vi "dfd_FXP Direct IIR II with IS.vi"(6 "state in":i64[](array[numeric]), 7 "quantizers":T5[](array[typedef]) {"source" items=["Coef a/k"=0, "Coef b/v"=7, "Input"=1, "Output"=2, "Multiplicand"=3, "Product"=4, "Sum"=5, "Delay"=6, "Gain"=8]}, 8 "filtering statistics in":T4(array[cluster]) {"statistics information"."min value" format="%.2f"; "statistics information"."max value" format="%.2f"; "Quantizer Source" items=["Coefficients a/k"=0, "Coefficients b/v"=7, "Input"=1, "Output"=2, "Multiplicand"=3, "Product"=4, "Sum"=5, "Delay"=6]}, 9 "coef a":T7, 10 "coef b":T7, 11 "X":T7) -> (0 "filtering statistics out":T4(array[cluster]) {"statistics information"."min value" format="%.2f"; "statistics information"."max value" format="%.2f"; "Quantizer Source" items=["Coefficients a/k"=0, "Coefficients b/v"=7, "Input"=1, "Output"=2, "Multiplicand"=3, "Product"=4, "Sum"=5, "Delay"=6]}, 3 "filtered X":T7, 4 "state out":i64[](array[numeric]))   [LabVIEW 2017, in "NI_DigFilter_FXP.lvlib"]
uses:
  <vilib>/addons/Digital Filter Design/NI_DigFilter_FXP.lvlib
  <vilib>/addons/Digital Filter Design/_Objects.llb/dfd_DFXP Data Type (vector).ctl
  <vilib>/addons/Digital Filter Design/_Objects.llb/dfd_DFXP Operation Parameter.ctl
  <vilib>/addons/Digital Filter Design/_Objects.llb/dfd_Internal Quantization Srcs.ctl
  <vilib>/addons/Digital Filter Design/_Objects.llb/DFD Quantization Sources.ctl
  <vilib>/addons/Digital Filter Design/_Objects.llb/DFD FXP Statistics Data.ctl
  <vilib>/addons/Digital Filter Design/_Objects.llb/dfd_DFXP Data Type (scaler).ctl
  <vilib>/addons/Digital Filter Design/NI_DigFilterLicensed.lvlib
panel:
  in  "DFXP Value":T1={"value"=0, "wl"=0, "iwl"=0, "Signed"=TRUE} {"value" format="%.0x"}
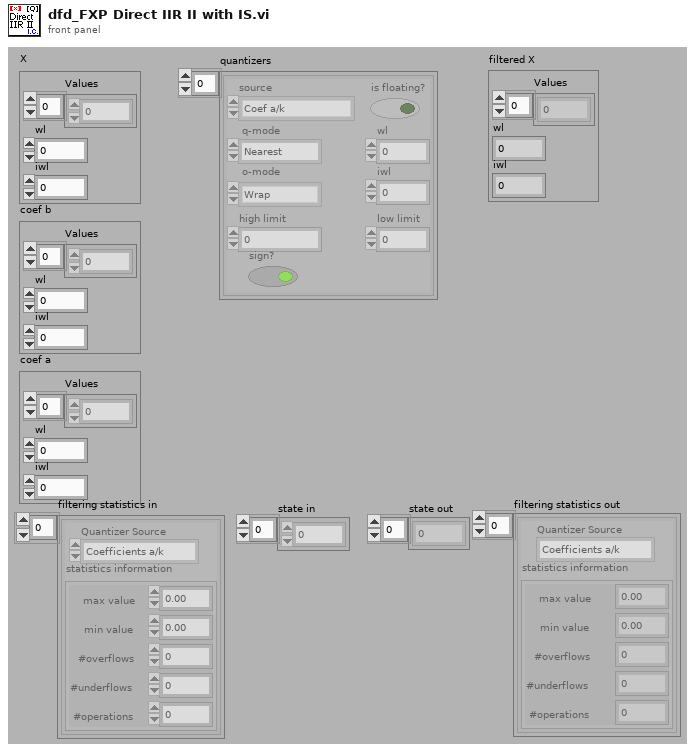
[diagram p1: front panel]
types:
  T1 = typedef "dfd_DFXP Data Type (scaler).ctl" = cluster{"value":i64, "wl":i16, "iwl":i16, "Signed":bool}
  T2 = typedef "NI_DigFilterLicensed.lvlib/DFD Quantization Sources.ctl" = u16
  T3 = typedef "NI_DigFilterLicensed.lvlib/DFD FXP Statistics Data.ctl" = cluster{"max value":ext, "min value":ext, "#overflows":i32, "#underflows":i32, "#operations":i32}
  T4 = cluster{"Quantizer Source":T2, "statistics information":T3}[]
  T5 = typedef "dfd_DFXP Operation Parameter.ctl" = cluster{"source":T6, "is floating?":bool, "o-mode":enum16{"Saturation", "Wrap"}, "q-mode":enum16{"Nearest", "Truncation"}, "wl":i16, "high limit":i64, "low limit":i64, "iwl":i16, "sign?":bool}
  T6 = typedef "NI_DigFilterLicensed.lvlib/dfd_Internal Quantization Srcs.ctl" = u16
  T7 = typedef "dfd_DFXP Data Type (vector).ctl" = cluster{"Values":i64[], "wl":i16, "iwl":i16}
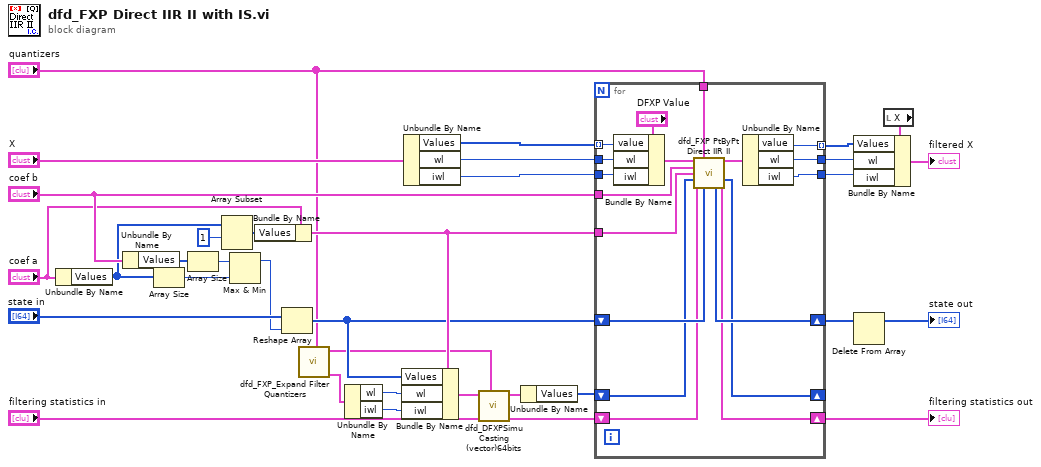
[diagram p0: block diagram]
diagram:
  n1 = Unbundle By Name("coef a") -> ("Values"=w21:i64[])
  n2 = Unbundle By Name("coef b") -> ("Values"=w22:i64[])
  n3 = Array Size(array=w21) -> (size(s)=w32:i32)
  n4 = Array Size(array=w22) -> (size(s)=w31:i32)
  n5 = Array Subset(array=w21, index=1) -> (w29:i64[])  [unwired: 1 in]
  n6 = Max & Min(x=w31, y=w32) -> (max(x,y)=w26:i32)  [unwired: 1 out]
  n7 = Bundle By Name(cluster="coef a", "Values"=w29) -> (w12:T7)
  n8 = Reshape Array("state in", w26) -> (w11:i64[])
  n9 = call <vilib>:"dfd_FXP_Expand Filter Quantizers.vi"("FXPOPs"="quantizers") -> ("Delay"=w9:T5, "Multiplicand"=w4:T5)  [unwired: 9 out]
  n10 = Unbundle By Name(w9) -> ("wl"=w8:i16, "iwl"=w7:i16)
  n11 = Bundle By Name(cluster=w12, "Values"=w11, "wl"=w8, "iwl"=w7) -> (w6:T7)
  n12 = Unbundle By Name("X") -> ("Values"=w19:i64[], "wl"=w18:i16, "iwl"=w17:i16)
  n13 = call <vilib>:"dfd_DFXPSimu Casting (vector)64bits.vi"("op params"=w4, "filtering statistics in"="filtering statistics in", "Value in"=w6) -> ("filtering statistics out"=w3:T4, "Value out"=w2:T7)  [unwired: 1 in, 6 out]
  n14 = Unbundle By Name(w2) -> ("Values"=w1:i64[])
  n15 = for {
    tunnel: w19 -> [w52] mode=indexing
    shift-right: [w47] -> w25
    shift-left: w11 -> [w48]
    tunnel: w12 -> [w37]
    tunnel: "coef b" -> [w49]
    tunnel: "quantizers" -> [w51]
    tunnel: [w40] -> w27 mode=indexing
    shift-right: [w45] -> w23
    shift-left: w3 -> [w46]
    tunnel: w18 -> [w42]
    tunnel: w17 -> [w41]
    tunnel: [w39] -> w14
    tunnel: [w38] -> w13
    shift-right: [w35] -> _
    shift-left: w1 -> [w36]
    n16 = Bundle By Name(cluster="DFXP Value", "value"=w52, "wl"=w42, "iwl"=w41) -> (w44:T1)
    n17 = call <vilib>:"dfd_FXP PtByPt Direct IIR II.vi"("x"=w44, "quantizers"=w51, "coef b[0..M]"=w49, "coef a[1..N]"=w37, "state tmp in"=w36, "filtering statistics in"=w46, "state in"=w48) -> ("filtered x"=w50:T1, "state tmp out"=w35:i64[], "state out"=w47:i64[], "filtering statistics out"=w45:T4)  [unwired: 5 out]
    n18 = Unbundle By Name(w50) -> ("value"=w40:i64, "wl"=w39:i16, "iwl"=w38:i16)
  }
  "filtering statistics out" <- w23
  n19 = Delete From Array(array=w25) -> (array with subset deleted=→"state out":i64[])  [unwired: 2 in, 1 out]
  n20 = local read "X"() -> (w15:T7)
  n21 = Bundle By Name(cluster=w15, "Values"=w27, "wl"=w14, "iwl"=w13) -> (→"filtered X":T7)
